vi "Create.vi"(8 "error in (no error)":errorcluster, 9 "Row":i32, 10 "Col Offset":i32, 11 "String":string) -> (0 "error out":errorcluster, 2 "Offset Past Symbol":i32, 3 "Number":refnum<class "Symbol.lvclass">)   [LabVIEW 2020, in "Symbol.lvclass"]
uses:
  Symbol.lvclass
  Symbol.lvclass/Symbol.ctl
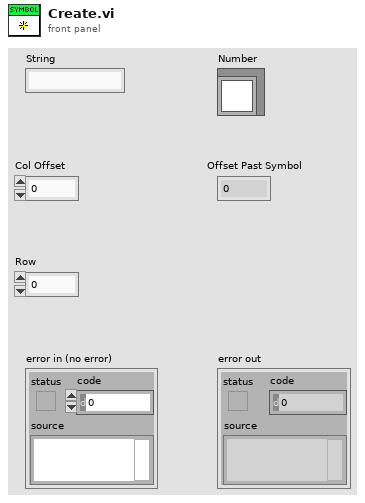
[diagram p1: front panel]
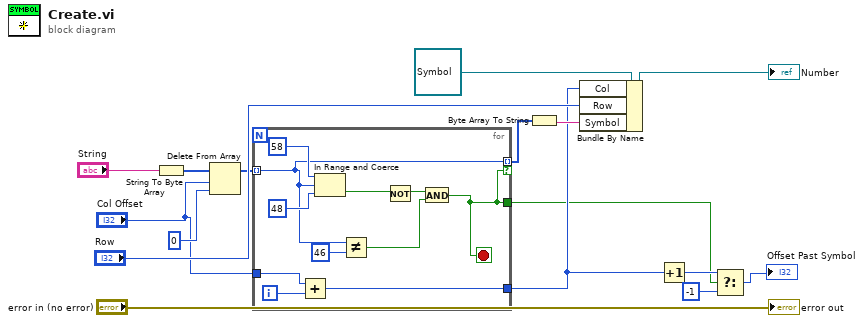
[diagram p0: block diagram]
diagram:
  n1 = String To Byte Array(string="String") -> (unsigned byte array=w11:u8[])
  n2 = Delete From Array(array=w11, length="Col Offset", index=0) -> (array with subset deleted=w10:u8[])  [unwired: 1 out]
  n3 = for {
    tunnel: w10 -> [w18] mode=indexing
    tunnel: "Col Offset" -> [w20]
    tunnel: [w19] -> w5
    tunnel: [w18] -> w6 mode=indexing if=w17
    tunnel: [w17] -> w2
    i -> [w21]
    stop <- w17 stop-if-true
    n4 = Add(x=w20, y=w21) -> (x+y=w19:i32)
    n5 = In Range and Coerce(upper limit=u8 58, x=w18, lower limit=u8 48) -> (In Range?=w25:bool)  [unwired: 1 out]
    n6 = Not Equal?(x=w18, y=u8 46) -> (x != y?=w22:bool)
    n7 = Not(x=w25) -> (.not. x?=w23:bool)
    n8 = And(x=w23, y=w22) -> (x .and. y?=w17:bool)
  }
  n9 = Byte Array To String(unsigned byte array=w6) -> (string=w7:string)
  n10 = Bundle By Name(cluster=refnum<class "Symbol.lvclass"> refnum ("Number"), "Col"=w5, "Row"="Row", "Symbol"=w7) -> (→"Number":refnum<class "Symbol.lvclass">)
  n11 = Increment(x=w5) -> (x+1=w4:i32)
  n12 = Select(t=w4, s=w2, f=-1) -> (s? t:f=→"Offset Past Symbol":i32)
  "error out" <- "error in (no error)"
